vi "Laurel Check Zero Reset.vi"(6 "Connection Type":T1, 8 "error in (no error)":errorcluster, 9 "All Items Byte Count (Flow Rate)":i32, 10 "TCP Network Connection in":refnum<k5>, 11 "VISA Refnum in":refnum<visa-resource-name>) -> (0 "error out":errorcluster, 1 "Stop Loop?":bool, 2 "TCP Network Connection out":refnum<k5>, 3 "VISA Refnum out":refnum<visa-resource-name>)   [LabVIEW 2019]
uses:
  Type Definitions/Laurel Connection Type.ctl
  Type Definitions/Laurel Serial Commands.ctl
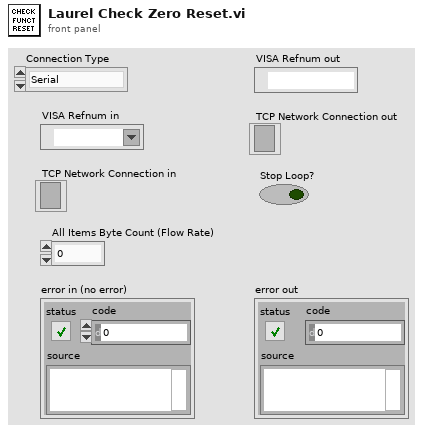
[diagram p1: front panel]
types:
  T1 = typedef "Laurel Connection Type.ctl" = enum16{"Serial", "TCP"}
  T2 = typedef "Laurel Serial Commands.ctl" = string
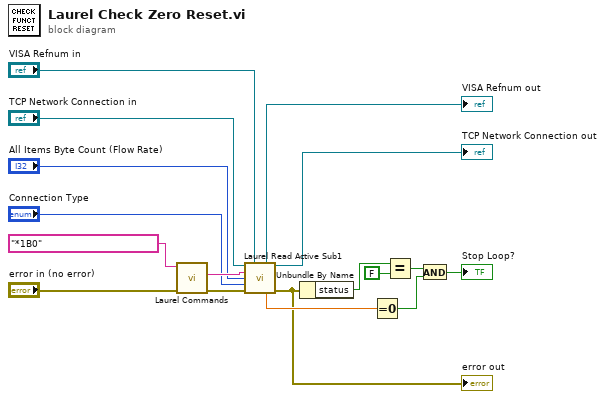
[diagram p0: block diagram]
diagram:
  n1 = call "Laurel Commands.vi"("Error In"="error in (no error)", "Laurel Serial Commands"=T2 "*1B0") -> ("Error Out"=w10:errorcluster, "Send Command out"=w11:string)  [unwired: 8 in]
  n2 = call "Laurel Read Active Sub1.vi"("TCP Network Connection in"="TCP Network Connection in", "Serial VISA"="VISA Refnum in", "Send Command in"=w11, "All Items Byte Count (Flow Rate)"="All Items Byte Count (Flow Rate)", "Connection Type"="Connection Type", "error in (no error)"=w10) -> ("VISA resource name 2"=→"VISA Refnum out":refnum<visa-resource-name>, "TCP Network Connection out"=→"TCP Network Connection out":refnum<k5>, "Gallons (Item 2)"=w13:dbl, "error out"=w8:errorcluster)  [unwired: 3 in, 3 out]
  "error out" <- w8
  n3 = Unbundle By Name(w8) -> ("status"=w14:bool)
  n4 = Equal To 0?(x=w13) -> (x = 0?=w17:bool)
  n5 = Equal?(x=w14, y=FALSE) -> (x = y?=w16:bool)
  n6 = And(x=w16, y=w17) -> (x .and. y?=→"Stop Loop?":bool)
